vi "Change Status.vi"(8 "error in (no error)":errorcluster, 10 "Value":T1(ring), 11 "Python Protocol in":refnum<class "Python Protocol.lvclass">) -> (0 "error out":errorcluster, 3 "Python Protocol out":refnum<class "Python Protocol.lvclass">)   [LabVIEW 2012, in "Python Protocol Actor.lvlib" / "Python Protocol.lvclass"]
uses:
  Python Protocol.lvclass
  Python Protocol.lvclass/Python Protocol.ctl
  Read State.vi
  Read Code.vi
  Read New.vi
  Read Open.vi
  Read Save.vi
  Read Refresh.vi
  Read Compiler.vi
  Read Start Time.vi
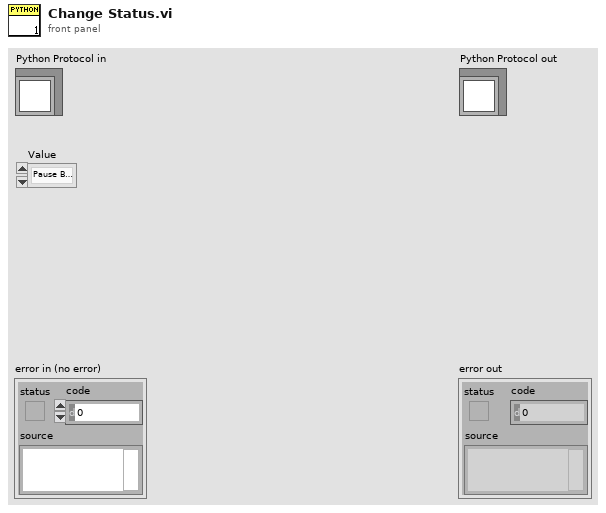
[diagram p1: front panel]
types:
  T1 = enum32{"Pause Button", "Play Button", "Media Stop Button"}
  T2 = enum8{"Enabled", "Disabled", "Disabled and Grayed Out"}
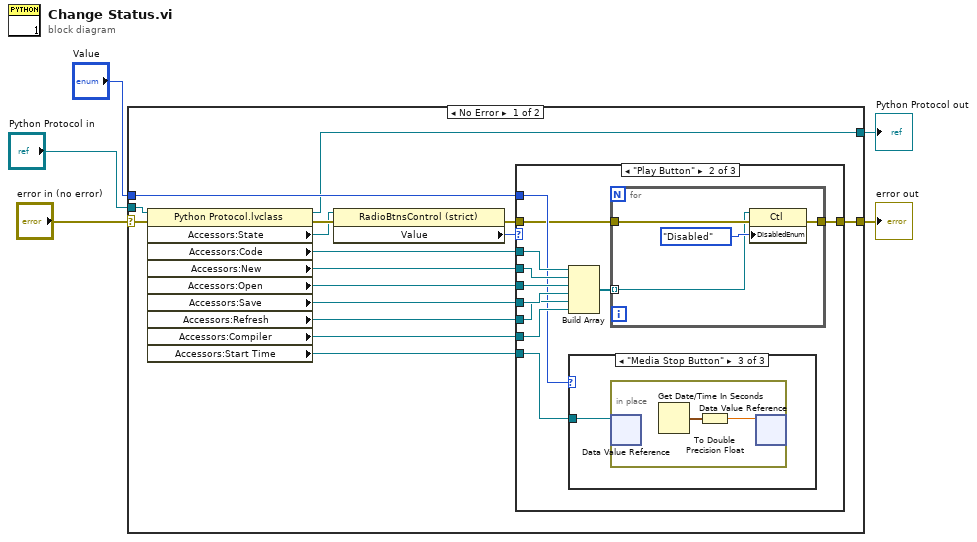
[diagram p0: block diagram]
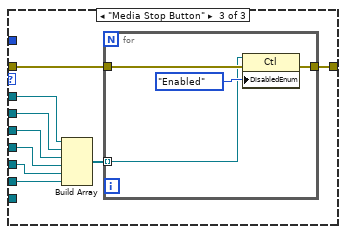
[diagram p5: hidden frame]
diagram:
  n1 = case shown="No Error" "error in (no error)" {
    selector: "error in (no error)" -> [w11 w55]
    tunnel: [w12 w55] -> w4
    tunnel: [w8 w54] -> w2
    tunnel: "Python Protocol in" -> [w19 w54]
    tunnel: "Value" -> [w9 _]
    frame No Error {
      n2 = property class="Python Protocol.lvclass"(reference=w19, error in=w11) -> (reference out=w8:refnum<class "Python Protocol.lvclass">, error out=w13:errorcluster, "Accessors:State"=w7:refnum<vi>, "Accessors:Code"=w10:refnum<vi>, "Accessors:New"=w18:refnum<vi>, "Accessors:Open"=w17:refnum<vi>, "Accessors:Save"=w16:refnum<vi>, "Accessors:Refresh"=w15:refnum<vi>, "Accessors:Compiler"=w14:refnum<vi>, "Accessors:Start Time"=w6:refnum<data-value>)
      n3 = property class="RadioBtnsControl (strict)"(reference=w7, error in=w13) -> (error out=w21:errorcluster, "Value"=w20:T1)  [unwired: 1 out]
      n4 = case shown="\"Play Button\"" w20 {
        tunnel: [w22 w27 w41] -> w12
        tunnel: w21 -> [w22 w24 w42]
        tunnel: w14 -> [_ w29 w43]
        tunnel: w18 -> [_ w33 w47]
        tunnel: w17 -> [_ w32 w46]
        tunnel: w16 -> [_ w31 w45]
        tunnel: w15 -> [_ w30 w44]
        tunnel: w10 -> [_ w26 w48]
        tunnel: w9 -> [_ w25 _]
        tunnel: w6 -> [_ w23 _]
        frame "Pause Button", Default {
        }
        frame "Play Button" {
          n5 = Build Array(w26, w33, w32, w31, w30, w29) -> (w28:refnum<vi>[])
          n6 = case shown="\"Media Stop Button\"" w25 {
            tunnel: w23 -> [_ _ w34]
            frame "Pause Button", Default {
            }
            frame "Play Button" {
            }
            frame "Media Stop Button" {
              n7 = in-place {
                n8 = in-place-dvr #1(w34) -> ()  [unwired: 2 out]
                n9 = Get Date/Time In Seconds() -> (seconds since 1Jan1904=w36:timestamp)
                n10 = To Double Precision Float(number=w36) -> (double precision float=w35:dbl)
                n11 = in-place-dvr #1(w35) -> ()  [unwired: 2 out]
              }
            }
          }
          n12 = for {
            tunnel: w24 -> [w39]
            tunnel: [w38] -> w27
            tunnel: w28 -> [w37] mode=indexing
            n13 = property class="Ctl"(reference=w37, error in=w39, "DisabledEnum"=T2."Disabled" ("Disabled")) -> (error out=w38:errorcluster)  [unwired: 1 out]
          }
        }
        frame "Media Stop Button" {
          n14 = Build Array(w48, w47, w46, w45, w44, w43) -> (w49:refnum<vi>[])
          n15 = for {
            tunnel: w42 -> [w52]
            tunnel: [w51] -> w41
            tunnel: w49 -> [w50] mode=indexing
            n16 = property class="Ctl"(reference=w50, error in=w52, "DisabledEnum"=T2."Enabled" ("Disabled")) -> (error out=w51:errorcluster)  [unwired: 1 out]
          }
        }
      }
    }
    frame Error {
    }
  }
  "error out" <- w4
  "Python Protocol out" <- w2
